vi "Read Report Folder.vi"(8 "error in (no error)":errorcluster, 11 "Project Action in":refnum<class "Project Action.lvclass">) -> (0 "error out":errorcluster, 2 "Report Folder":path, 3 "Project Action out":refnum<class "Project Action.lvclass">)   [LabVIEW 2020, in "ProjectBuilder.lvlib" / "Project Action.lvclass"]
uses:
  Project Action.lvclass
  Project Action.lvclass/Project Action.ctl
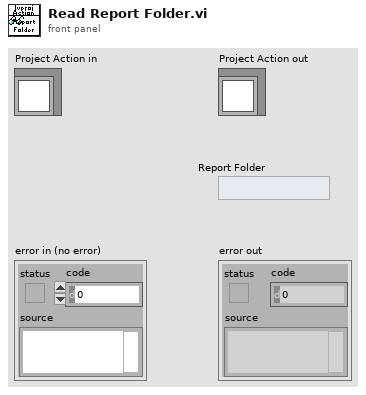
[diagram p1: front panel]
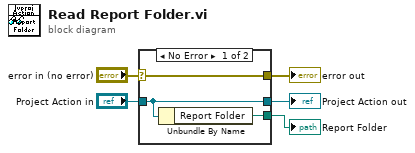
[diagram p0: block diagram]
diagram:
  n1 = case shown="No Error" "error in (no error)" {
    selector: "error in (no error)" -> [w8 w9]
    tunnel: [w8 w9] -> w4
    tunnel: [w7 w10] -> w2
    tunnel: "Project Action in" -> [w7 w10]
    tunnel: [w6 _] -> w1
    frame No Error {
      n2 = Unbundle By Name(w7) -> ("Report Folder"=w6:path)
    }
    frame Error {
    }
  }
  "error out" <- w4
  "Project Action out" <- w2
  "Report Folder" <- w1
